vi "Remove Single String Array.vi"(11 "Close in":string[](array[string])) -> (3 "Close out":string[](array[string]))   [LabVIEW 2016, in "SLSC Switch.lvlib" / "SLSC Switch.lvclass"]
uses:
  SLSC Switch.lvclass
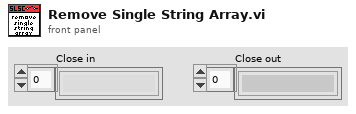
[diagram p1: front panel]
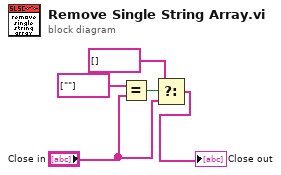
[diagram p0: block diagram]
diagram:
  n1 = Equal?(x=string[] [""], y="Close in") -> (x = y?=w2:bool)
  n2 = Select(t=string[] [], s=w2, f="Close in") -> (s? t:f=→"Close out":string[])
